vi "ConfigureScanTrigger.vi"(8 "Error In":errorcluster, 10 "Scan Configuration":T1, 11 "Keithley 7001 In":refnum<visa-resource-name>) -> (0 "Error Out":errorcluster, 3 "Keithley 7001 Out":refnum<visa-resource-name>)   [LabVIEW 2012]
uses:
  TriggerScanConfiguration.ctl
  driver/Public/Controls/ScanSource.ctl
  driver/Keithley-7001.lvlib
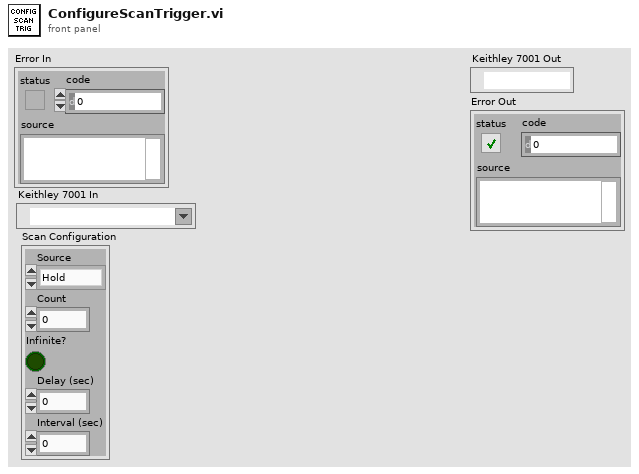
[diagram p1: front panel]
types:
  T1 = typedef "TriggerScanConfiguration.ctl" = cluster{"Source":T2, "Count":u32, "Infinite?":bool, "Delay (sec)":dbl, "Interval (sec)":dbl}
  T2 = typedef "Keithley-7001.lvlib/ScanSource.ctl" = enum16{"Hold", "Immediate", "Timer", "Manual", "Bus", "TLink", "External"}
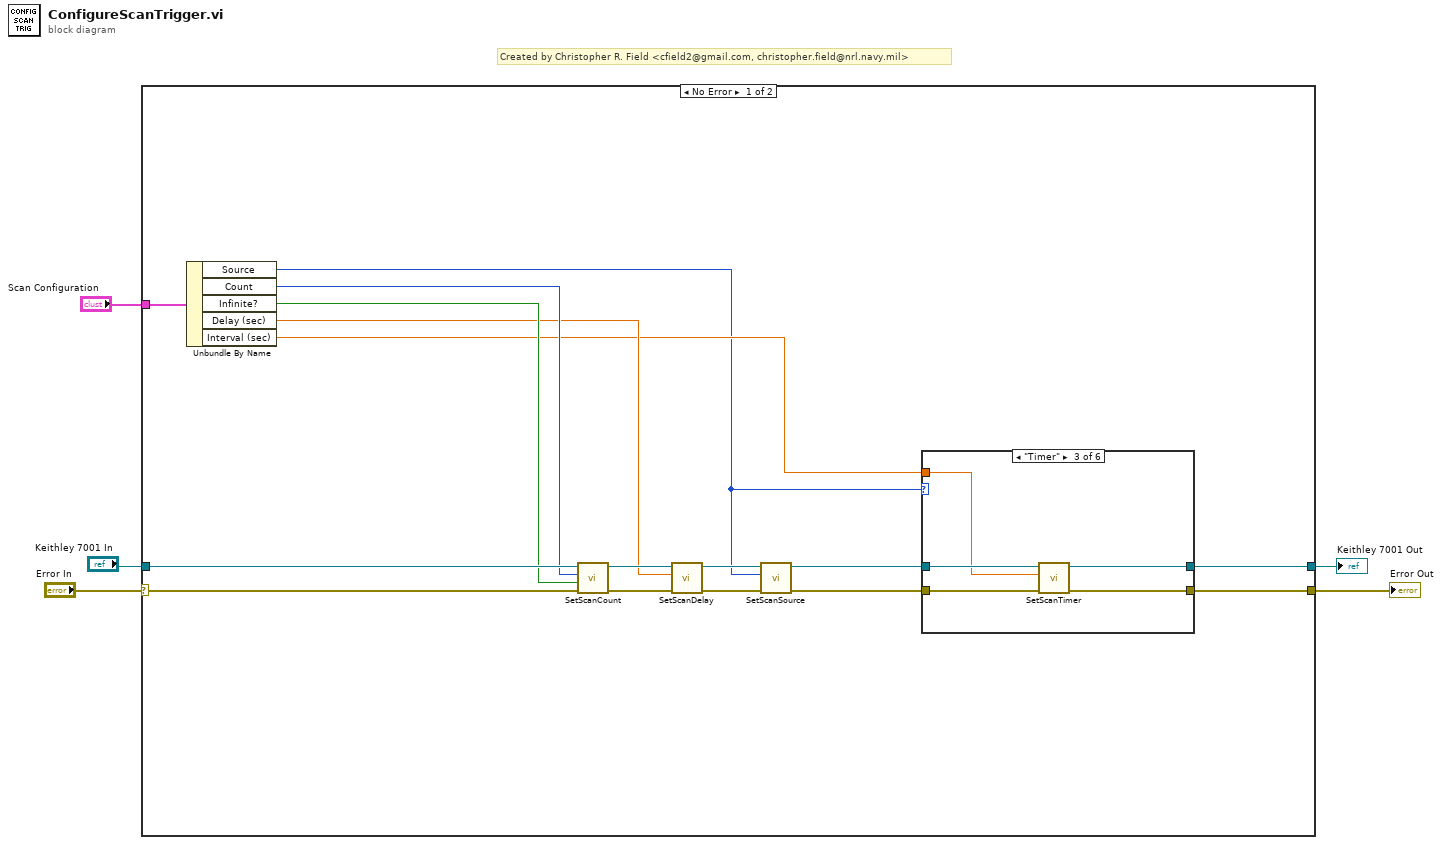
[diagram p0: block diagram]
diagram:
  # "Created by Christopher R. Field <cfield2@gmail.com, christopher.field@nrl.navy.mil>"
  n1 = case shown="No Error" "Error In" {
    selector: "Error In" -> [w15 w37]
    tunnel: "Keithley 7001 In" -> [w14 w38]
    tunnel: [w13 w38] -> w3
    tunnel: [w12 w37] -> w2
    tunnel: "Scan Configuration" -> [w11 _]
    frame No Error {
      n2 = Unbundle By Name(w11) -> ("Source"=w6:T2, "Count"=w10:u32, "Infinite?"=w9:bool, "Delay (sec)"=w8:dbl, "Interval (sec)"=w7:dbl)
      n3 = call "SetScanCount.vi"("Error In"=w15, "Infinite?"=w9, "Count (1-9999)"=w10, "Keithley 7001 In"=w14) -> ("Error Out"=w20:errorcluster, "Keithley 7001 Out"=w21:refnum<visa-resource-name>)  [unwired: 6 in]
      n4 = call "SetScanDelay.vi"("Error In"=w20, "Delay (sec)"=w8, "Keithley 7001 In"=w21) -> ("Error Out"=w19:errorcluster, "Keithley 7001 Out"=w18:refnum<visa-resource-name>)  [unwired: 7 in]
      n5 = call "SetScanSource.vi"("Error In"=w19, "Scan Source"=w6, "Keithley 7001 In"=w18) -> ("Error Out"=w17:errorcluster, "Keithley 7001 Out"=w16:refnum<visa-resource-name>)  [unwired: 7 in]
      n6 = case shown="\"Timer\"" w6 {
        tunnel: w17 -> [w22 w24 w29 w31 w33 w35]
        tunnel: w16 -> [w23 w25 w30 w32 w34 w36]
        tunnel: [w23 w25 w27 w32 w34 w36] -> w13
        tunnel: [w22 w24 w28 w31 w33 w35] -> w12
        tunnel: w7 -> [_ _ w26 _ _ _]
        frame "Hold", Default {
        }
        frame "Immediate" {
        }
        frame "Timer" {
          n7 = call "SetScanTimer.vi"("Error In"=w29, "Interval (sec)"=w26, "Keithley 7001 In"=w30) -> ("Error Out"=w28:errorcluster, "Keithley 7001 Out"=w27:refnum<visa-resource-name>)  [unwired: 7 in]
        }
        frame "Manual" {
        }
        frame "Bus" {
        }
        frame "External" {
        }
      }
    }
    frame Error {
    }
  }
  "Keithley 7001 Out" <- w3
  "Error Out" <- w2
